vi "GUI_FilterWheels.vi"() -> ()   [LabVIEW 2020]
uses:
  Device Drivers/FilterWheels/posTypDef.ctl
  Device Drivers/FilterWheels/ModeTypDEf.ctl
panel:
  out "reference out":refnum<vi>
  out "#ofChannels":i32
  out "indecator ref array":refnum<vi>[](array[refnum])
  in  "time to wait (TCP) 2":i32=10
  in  "plot":bool=TRUE
  out "ratio(h)":bool
  out "fixsize":bool
  in  "shotnumber":i32
  out "error (h)":bool
  out "Device Name (h)":string="StagingDG645 1"
  in  "Main Tap":T1(tab)
  out "Description":string[](array[string])
  in  "ModeAll":T2
  in  "modeArray":T2[](array[typedef])
  out "Status 2":u32[](array[colorbox])
  out "Name":string[](array[string])
  in  "pos":T3[](array[typedef])
  out "device status":string
  out "local Port":u16=65427
  out "port or service name":u16=65426
  out "Remote Host":string="192.168.11.97"
  in  "timeout ms (slow resp)":i32=500
  in  "reset":bool
  out "All Devices (h)":string[](array[string])=["StagingDG645 1", "StagingDG645 2"]
  in  "time to wait (TCP)":i32=10
  out "error out":errorcluster
  out "connections (hidden)":variant[](array[variant])=[variant(refnum<k16> refnum), variant(refnum<k16> refnum)]
  in  "time to wait (main loop)":i32=10
  out "Data String":string="Amplitude.Ch AB,3.000000000000\r\nAmplitude.Ch CD,4.000000000000\r\nAmplitude.Ch EF,4.000000000000\r\nAmplitude.Ch GH,4.000000000000\r\nAmplitude.Ch T0,4.000000000000\r\nDelay.Ch A,0.000000000000\r\nDelay.Ch B,0.030000000000\r\nDelay.Ch C,0.000000000000\r\nDelay.Ch D,0.030000000000\r\nDelay.Ch E,0.000000000000\r\nDelay.Ch F,0.030000000000\r\nDelay.Ch G,0.000000000000\r\nDelay.Ch H,0.030000000000\r\nDelay.Ch T0,0.000000000000\r\nDelay.Ch T1,0.030000\r\nInhibit,Triggers\r\nLinked.Ch A,T0\r\nLinked.Ch B,A\r\nLinked.Ch C,T0\r\nLinked.Ch D,C\r\nLinked.Ch E,T0\r\nLinked.Ch F,E\r\nLinked.Ch G,T0\r\nLinked.Ch H,G\r\nLocalSavingPath,c:\\temp\r\nSave,off\r\nTrigger.ExecuteSingleShot,\r\nTrigger.Level,1.000000\r\nTrigger.Rate,10.000000\r\nTrigger.Source,External rising edges\r\ntimeout,0.000000\r\nPolarity.Ch AB,Positive\r\nPolarity.Ch CD,Positive\r\nPolarity.Ch EF,Positive\r\nPolarity.Ch GH,Positive\r\nPolarity.Ch T0,Positive\r\n"
  in  "Local Saving Path":path
  out "concatenated string":string
  out "subscriberString":string
  out "error message":string
  out "new data":bool
  out "Data Connection out":bool=TRUE
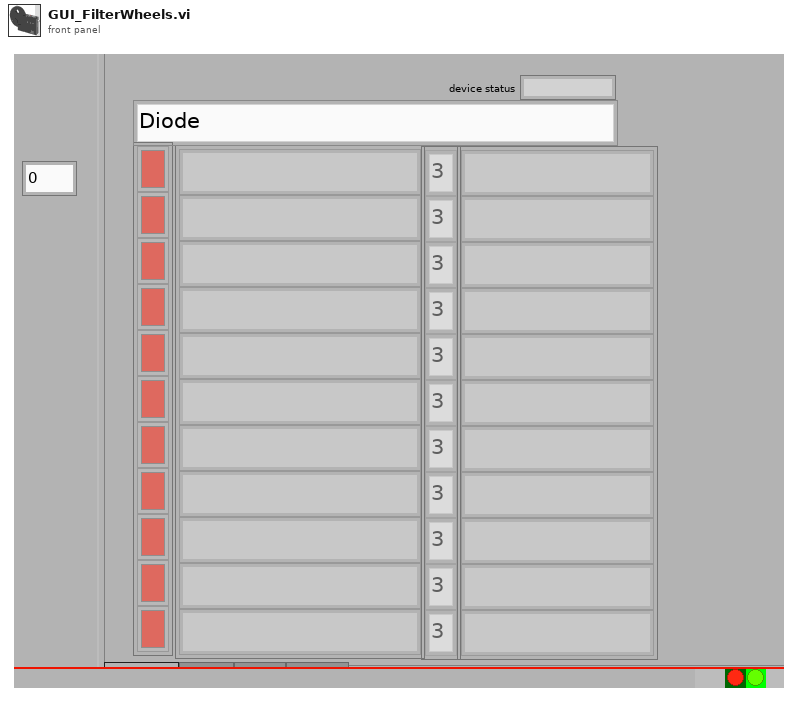
[diagram p1: front panel]
types:
  T1 = enum32{"All Channels", "Network", "Internal", "Advanced"}
  T2 = typedef "ModeTypDEf.ctl" = enum16{"Diode", "Low Power", "High Power", "undefined"}
  T3 = typedef "posTypDef.ctl" = enum16{"1", "2", "3", "4", "5", "6"}
  T4 = typedef "EventTypDef.ctl" = refnum<user-event>
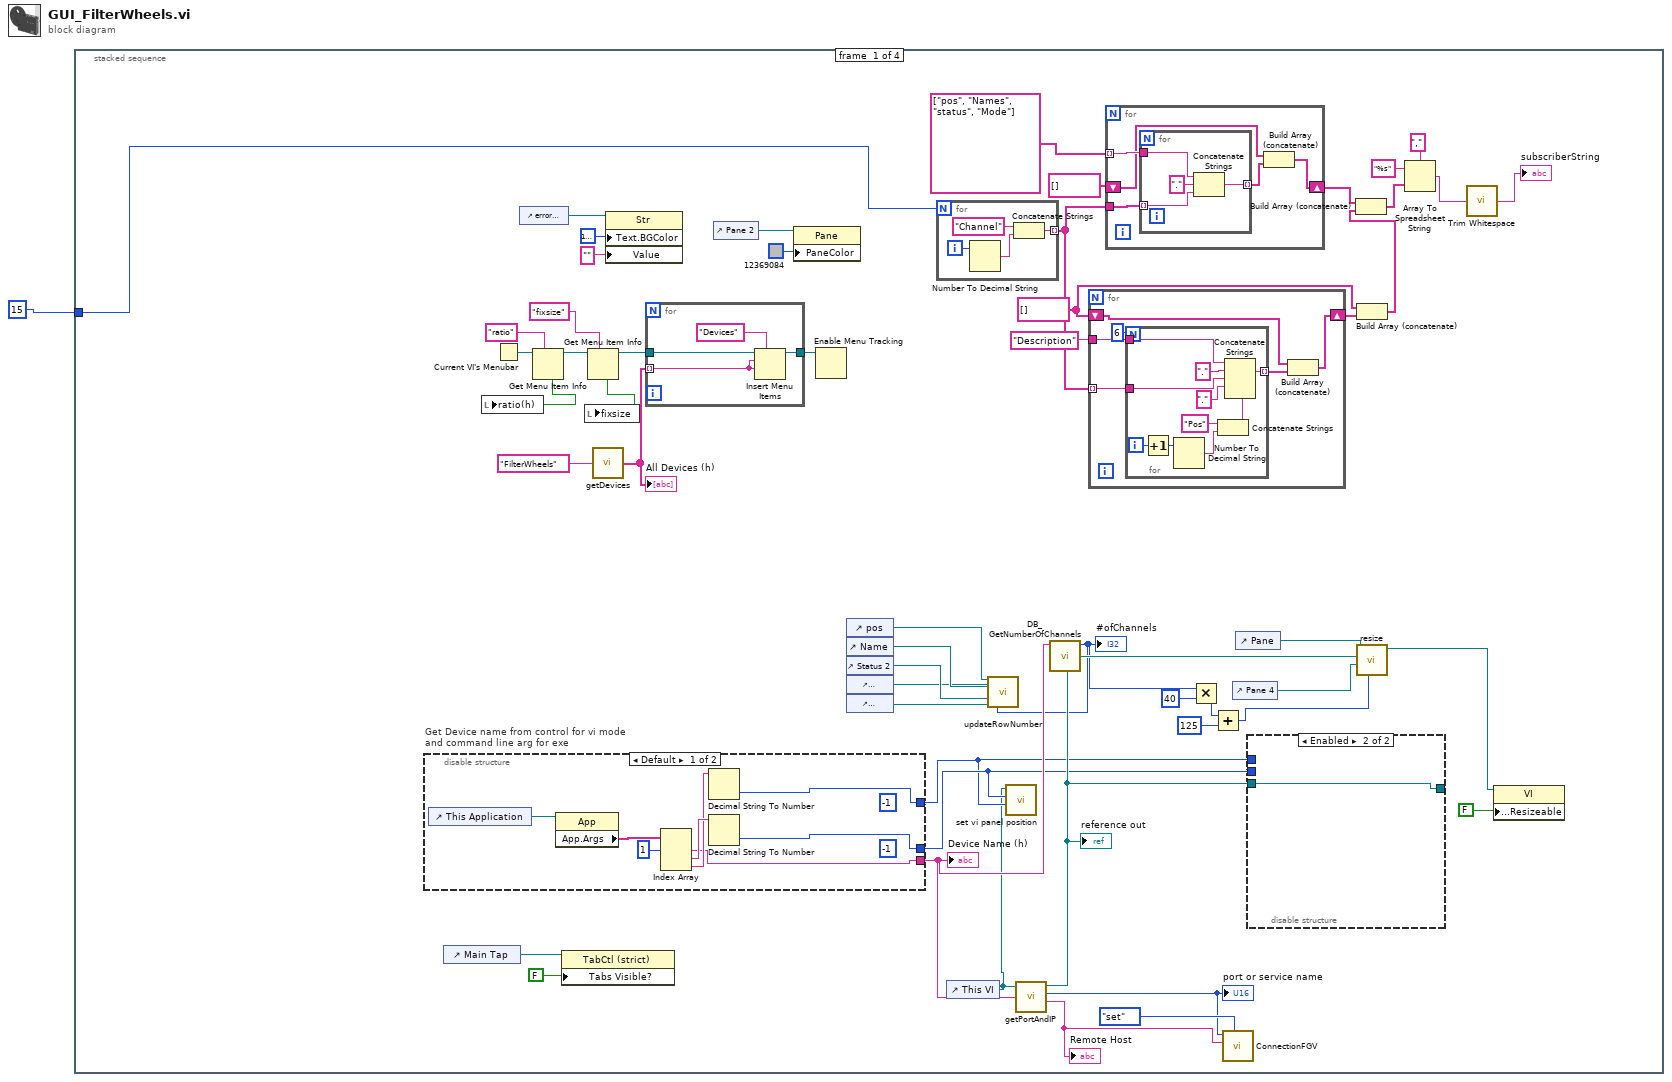
[diagram p0: block diagram]
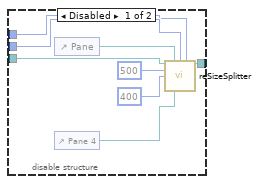
[diagram p2: hidden frame]
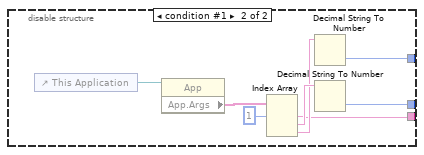
[diagram p3: hidden frame]
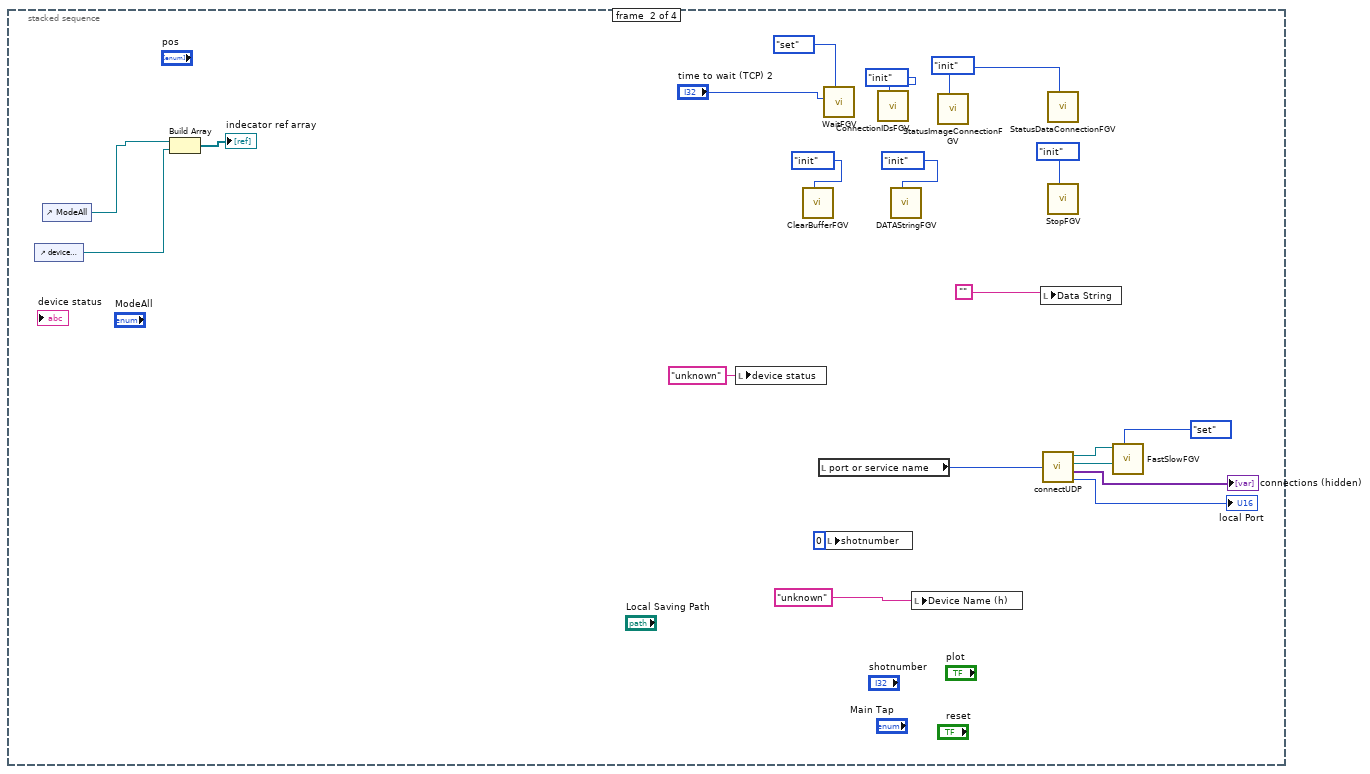
[diagram p4: hidden frame]
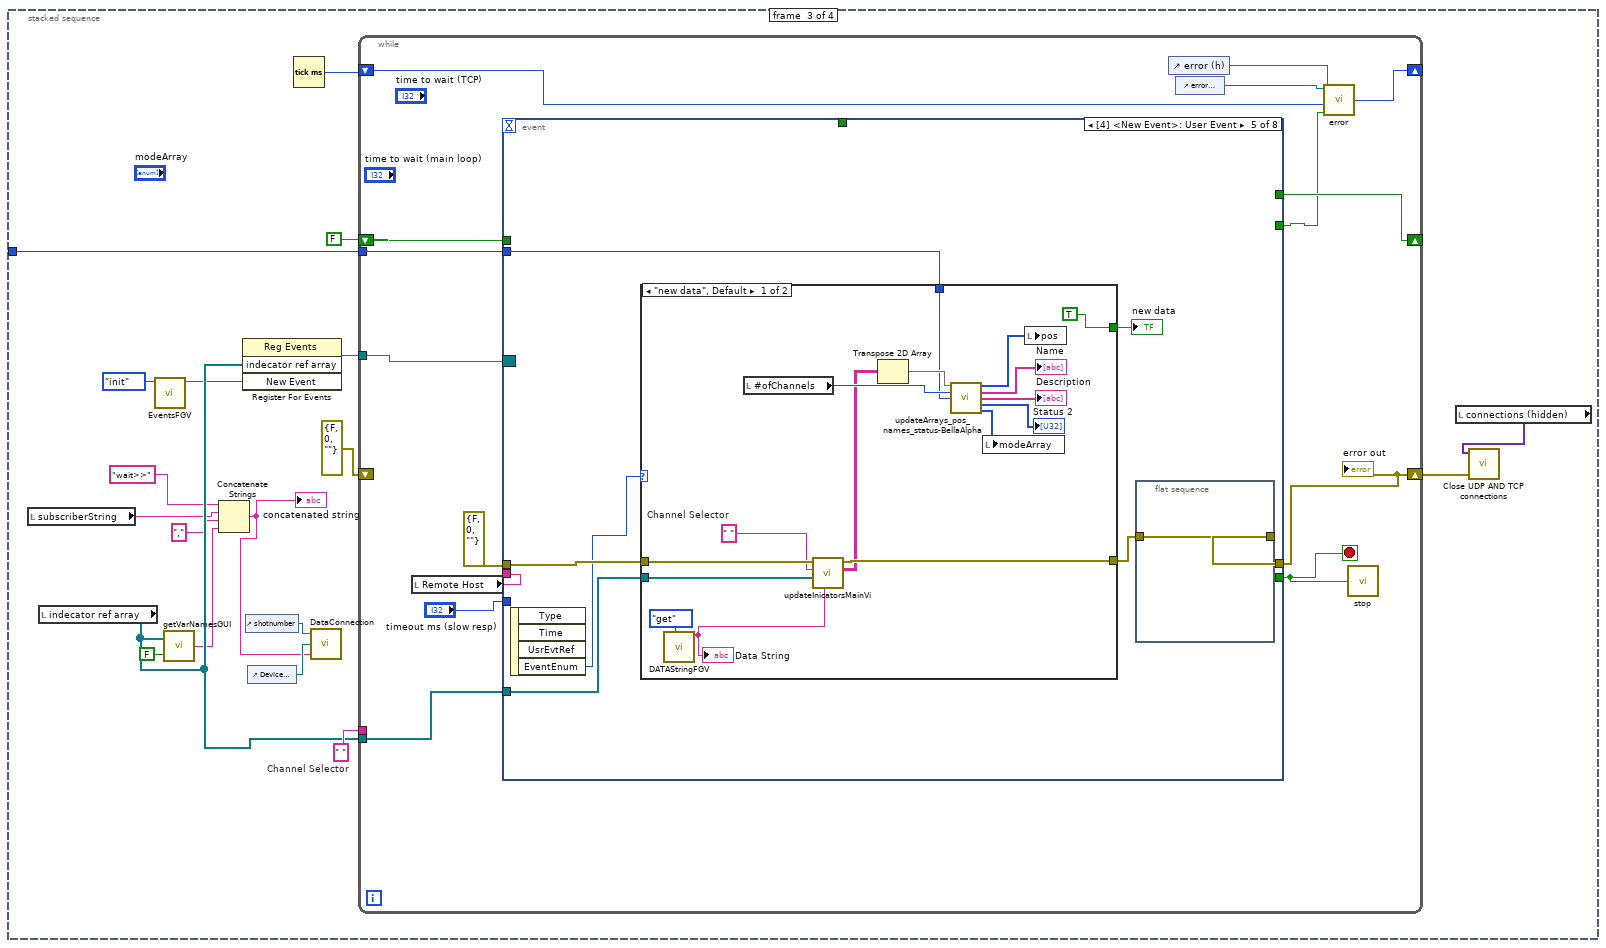
[diagram p5: hidden frame]
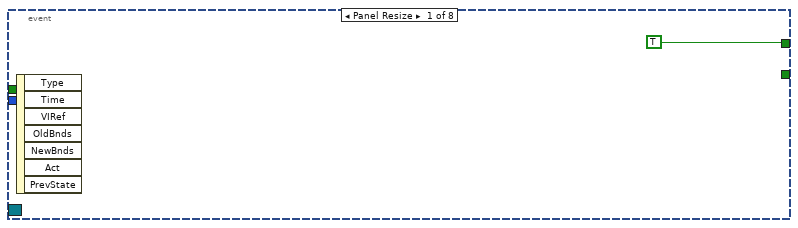
[diagram p6: hidden frame]
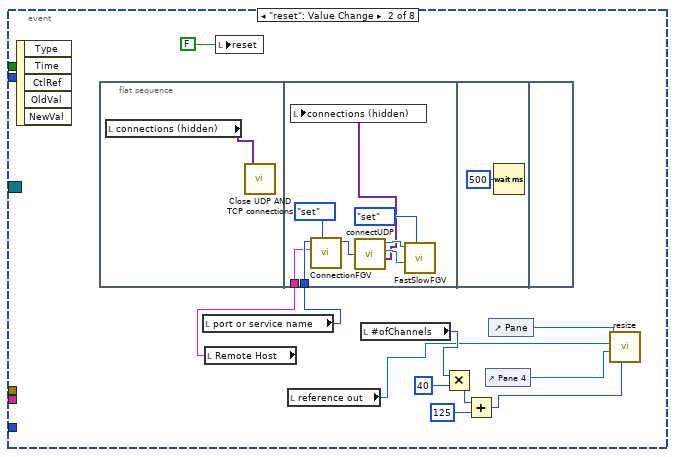
[diagram p7: hidden frame]
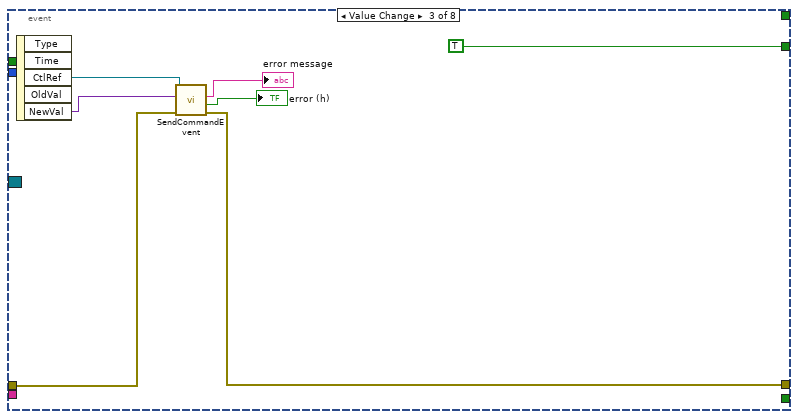
[diagram p8: hidden frame]
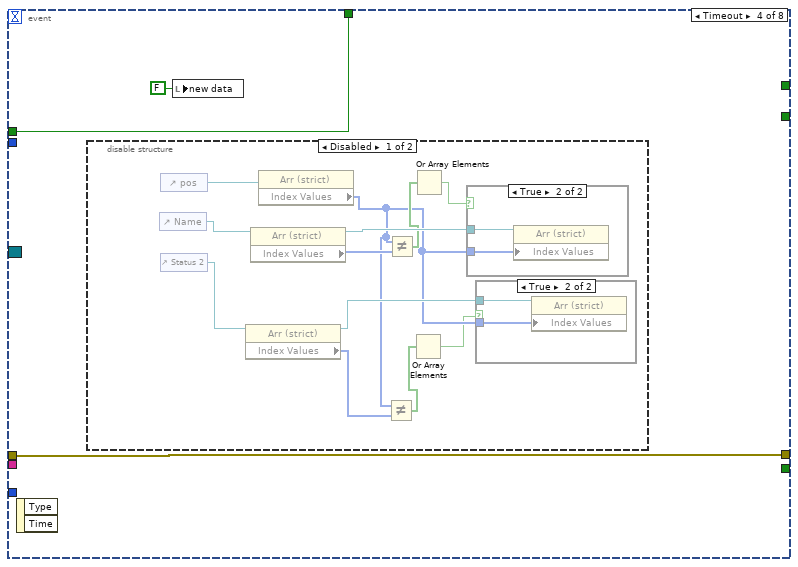
[diagram p9: hidden frame]
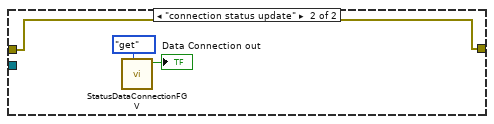
[diagram p13: hidden frame]
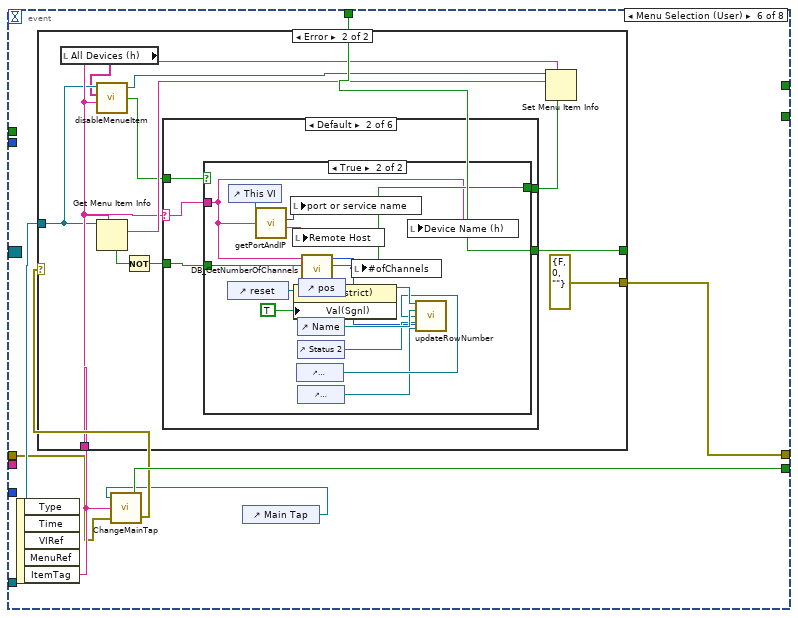
[diagram p14: hidden frame]
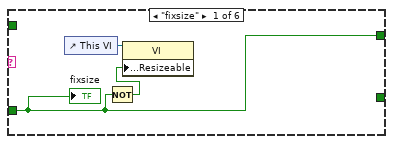
[diagram p16: hidden frame]
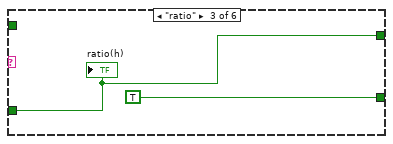
[diagram p18: hidden frame]
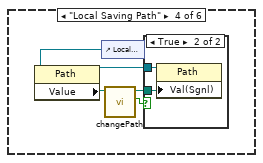
[diagram p19: hidden frame]
diagram:
  n1 = stacked-sequence {
    tunnel: 15 ("max channels") -> [w2 _ w133 _]
    frame #0 {
      w9 = string[] []
      n2 = disable-structure "Get Device name from control for vi mode\nand command line arg for exe" shown="Default" {
        disable-tunnel: [w97 w105] -> w33
        disable-tunnel: [w99 w108] -> w19
        disable-tunnel: [w100 w107] -> w18
        frame condition #0 (active) {
          (unwired) i16 -1 ("left")
          (unwired) i16 -1 ("left")
          n3 = control-ref of="This Application"() -> (w104:refnum<vi>)
          n4 = property class="App"(reference=w104) -> ("App.Args"=w98:string[])  [unwired: 1 in, 2 out]
          n5 = Index Array(array=w98, index #1=1 ("index")) -> (element #1=w97:string, element #2=w102:string, element #3=w101:string)  [unwired: 2 in]
          n6 = Decimal String To Number(string=w101) -> (number=w100:i32)  [unwired: 2 in, 1 out]
          n7 = Decimal String To Number(string=w102) -> (number=w99:i32)  [unwired: 2 in, 1 out]
        }
        frame condition #1 {
          n8 = control-ref of="This Application"() -> (w112:refnum<vi>)
          n9 = property class="App"(reference=w112) -> ("App.Args"=w106:string[])  [unwired: 1 in, 2 out]
          n10 = Index Array(array=w106, index #1=1 ("index")) -> (element #1=w105:string, element #2=w110:string, element #3=w109:string)  [unwired: 2 in]
          n11 = Decimal String To Number(string=w109) -> (number=w107:i32)  [unwired: 2 in, 1 out]
          n12 = Decimal String To Number(string=w110) -> (number=w108:i32)  [unwired: 2 in, 1 out]
        }
      }
      "Device Name (h)" <- w33
      n13 = control-ref of="Main Tap"() -> (w54:refnum<vi>)
      n14 = Current VI's Menubar() -> (w47:refnum<k9>)
      n15 = control-ref of="error message"() -> (w41:refnum<vi>)
      n16 = Get Menu Item Info(7:"ratio" ("item tag"), 11:w47) -> (3:w45:refnum<k9>, 4:w46:bool)  [unwired: 1 in, 5 out]
      n17 = local write "ratio(h)"(w46) -> ()
      n18 = property class="TabCtl (strict)"(reference=w54, "Tabs Visible?"=FALSE) -> ()  [unwired: 1 in, 2 out]
      n19 = Get Menu Item Info(7:"fixsize" ("item tag"), 11:w45) -> (3:w37:refnum<k9>, 4:w43:bool)  [unwired: 1 in, 5 out]
      n20 = local write "fixsize"(w43) -> ()
      n21 = call "getDevices.vi"("Device Class"="FilterWheels") -> ("All Devices"=w35:string[])
      "All Devices (h)" <- w35
      n22 = property class="Str"(reference=w41, "Text.BGColor"=u32 16777238, "Value"="") -> ()  [unwired: 1 in, 2 out]
      n23 = for {
        tunnel: w37 -> [w87]
        tunnel: [w86] -> w36
        tunnel: w35 -> [w84] mode=indexing
        n24 = Insert Menu Items(5:"Devices" ("menu tag"), 7:w84, 8:w84, 9:w87) -> (3:w86:refnum<k9>)  [unwired: 2 in, 2 out]
      }
      n25 = control-ref of="Pane 2"() -> (w39:refnum<vi>)
      n26 = property class="Pane"(reference=w39, "PaneColor"=u32 12369084) -> ()  [unwired: 1 in, 2 out]
      n27 = Enable Menu Tracking(4:w36) -> ()  [unwired: 2 in, 2 out]
      n28 = control-ref of="pos"() -> (w28:refnum<vi>)
      n29 = control-ref of="Name"() -> (w27:refnum<vi>)
      n30 = control-ref of="Status 2"() -> (w26:refnum<vi>)
      n31 = control-ref of="modeArray"() -> (w23:refnum<vi>)
      n32 = control-ref of="Description"() -> (w10:refnum<vi>)
      n33 = for {
        N: w2 -> [_]
        tunnel: [w80] -> w6 mode=indexing
        i -> [w83]
        n34 = Number To Decimal String(number=w83) -> (decimal integer string=w81:string)  [unwired: 1 in]
        n35 = Concatenate Strings("Channel" ("string"), w81) -> (w80:string)
      }
      n36 = control-ref of="This VI"() -> (w17:refnum<vi>)
      n37 = call "set vi panel position.vi"("top"=w18, "left"=w19, "This VI"=w17) -> ()  [unwired: 7 in, 2 out]
      n38 = call "getPortAndIP.vi"("Device Name"=w33, "This Vi"=w17) -> ("Remote Host"=w50:string, "port or service name"=w49:u16, "reference out"=w22:refnum<vi>)  [unwired: 2 in, 2 out]
      "port or service name" <- w49
      "Remote Host" <- w50
      "reference out" <- w22
      n39 = call "DB_GetNumberOfChannels.vi"("DeviceName"=w33) -> ("Numeric"=w20:i32)  [unwired: 9 in, 1 out]
      "#ofChannels" <- w20
      n40 = call "updateRowNumber.vi"("Array in"=w28, "Name"=w27, "modeArray 2"=w23, "Status 3"=w26, "Description"=w10, "No of channels"=w20) -> ()  [unwired: 10 in]
      n41 = for {
        tunnel: w6 -> [w59] mode=indexing
        tunnel: "Description" ("string") -> [w60]
        shift-right: [w55] -> w7
        shift-left: w9 -> [w57]
        n42 = for {
          N: 6 -> [_]
          tunnel: w60 -> [w70]
          tunnel: w59 -> [w69]
          tunnel: [w68] -> w56 mode=indexing
          i -> [w62]
          n43 = Increment(x=w62) -> (x+1=w61:i32)
          n44 = Number To Decimal String(number=w61) -> (decimal integer string=w65:string)  [unwired: 1 in]
          n45 = Concatenate Strings("Pos" ("string"), w65) -> (w63:string)
          n46 = Concatenate Strings(w70, "." ("string"), w69, "." ("string"), w63) -> (w68:string)
        }
        n47 = Build Array (concatenate)(w57, w56) -> (w55:string[])
      }
      n48 = for {
        tunnel: string[] ["pos", "Names", "status", "Mode"] -> [w74] mode=indexing
        tunnel: w6 -> [w75]
        shift-right: [w72] -> w4
        shift-left: string[] [] -> [w71]
        n49 = for {
          tunnel: w75 -> [w77] mode=indexing
          tunnel: w74 -> [w79]
          tunnel: [w76] -> w73 mode=indexing
          n50 = Concatenate Strings(w79, "." ("string"), w77) -> (w76:string)
        }
        n51 = Build Array (concatenate)(w71, w73) -> (w72:string[])
      }
      n52 = Multiply(x=w20, y=40) -> (x*y=w11:i32)
      n53 = Add(x=w11, y=125) -> (x+y=w12:i32)
      n54 = call "ConnectionFGV.vi"("command"=enum16{"get", "set", "init"}."set", "Remote Host in"=w50, "port or service name in"=w49) -> ()  [unwired: 7 in, 2 out]
      n55 = control-ref of="Pane 4"() -> (w15:refnum<vi>)
      n56 = control-ref of="Pane"() -> (w16:refnum<vi>)
      n57 = disable-structure shown="Enabled" {
        disable-tunnel: w19 -> [w94 _]
        disable-tunnel: w18 -> [w93 _]
        disable-tunnel: w22 -> [w91 w96]
        disable-tunnel: [w88 w96] -> _
        frame Disabled {
          n58 = control-ref of="Pane"() -> (w95:refnum<vi>)
          n59 = control-ref of="Pane 4"() -> (w92:refnum<vi>)
          n60 = call "reSizeSplitter.vi"("this vi"=w91, "pane"=w95, "left"=w94, "top"=w93, "Width"=u32 500, "Height"=u32 400, "pane2"=w92) -> ("reference out"=w88:refnum<vi>)  [unwired: 8 in]
        }
        frame Enabled {
        }
      }
      n61 = Build Array (concatenate)(w9, w7) -> (w5:string[])
      n62 = Build Array (concatenate)(w4, w5) -> (w3:string[])
      n63 = call "resize.vi"("Height"=w12, "Pane 4"=w15, "reference out 2"=w22, "Pane in"=w16) -> ("reference out"=w21:refnum<vi>)  [unwired: 7 in]
      n64 = Array To Spreadsheet String(delimiter (Tab)=",", array=w3, 3:"%s" ("format string")) -> (spreadsheet string=w25:string)
      n65 = call <vilib>:"Trim Whitespace.vi"("string"=w25) -> ("trimmed string"=→"subscriberString":string)  [unwired: 1 in]
      n66 = property class="VI"(reference=w21, "Front Panel.Resizeable"=FALSE ("Front Panel Window:Resizable")) -> ()  [unwired: 1 in, 2 out]
    }
    frame #1 {
      w125 = enum16{"get", "set", "init"}."init" ("Command")
      n67 = control-ref of="device status"() -> (w114:refnum<vi>)
      n68 = control-ref of="ModeAll"() -> (w115:refnum<vi>)
      n69 = Build Array(w115, w114) -> (→"indecator ref array":refnum<vi>[])
      n70 = local write "device status"("unknown" ("device status")) -> ()
      n71 = call "ClearBufferFGV.vi"("Command"=enum16{"set", "get", "init"}."init") -> ()  [unwired: 10 in, 1 out]
      n72 = local read "port or service name"() -> (w121:u16)
      n73 = call "WaitFGV.vi"("Command"=enum16{"get", "set", "init"}."set", "milliseconds to wait"="time to wait (TCP) 2") -> ()  [unwired: 9 in, 1 out]
      n74 = local write "shotnumber"(0 ("shotnumber")) -> ()
      n75 = call "ConnectionIDsFGV.vi"("Command"=enum16{"add", "get", "init"}."init") -> ()  [unwired: 10 in, 1 out]
      n76 = call "DATAStringFGV.vi"("Command"=enum16{"get", "set", "init"}."init") -> ()  [unwired: 9 in, 2 out]
      n77 = local write "Device Name (h)"("unknown" ("Device Name")) -> ()
      n78 = call "StatusImageConnectionFGV.vi"("Command"=w125) -> ()  [unwired: 10 in, 1 out]
      n79 = local write "Data String"("") -> ()
      n80 = call "connectUDP.vi"("port or service name NOT USED"=w121) -> ("fast ID (h)"=w120:refnum<k16>, "slow ID (h)"=w119:refnum<k16>, "connections (hidden)"=→"connections (hidden)":variant[], "local Port"=→"local Port":u16)
      n81 = call "StatusDataConnectionFGV.vi"("Command"=w125) -> ()  [unwired: 10 in, 1 out]
      n82 = call "StopFGV.vi"("Command"=enum16{"set", "get", "init"}."init") -> ()  [unwired: 9 in, 2 out]
      n83 = call "FastSlowFGV.vi"("Command"=enum16{"get", "set", "init"}."set", "slow ID"=w119, "fast ID"=w120) -> ()  [unwired: 7 in, 2 out]
    }
    frame #2 {
      w143 = " "  # Channel Selector
      n84 = local read "subscriberString"() -> (w138:string)
      n85 = local read "indecator ref array"() -> (w142:refnum<vi>[])
      n86 = call "EventsFGV.vi"("Command"=enum16{"get", "init"}."init") -> ("New Event"=w135:T4)  [unwired: 9 in, 1 out]
      n87 = call "getVarNamesGUI.vi"("start"=FALSE, "Array"=w142) -> ("String"=w137:string)
      n88 = Concatenate Strings("wait>>" ("string"), w138, "," ("string"), w137) -> (w140:string)
      "concatenated string" <- w140
      n89 = register-events(w142, w135) -> (reference out=w144:refnum<event-registration>)  [unwired: 2 in, 1 out]
      n90 = control-ref of="shotnumber"() -> (w146:refnum<vi>)
      n91 = control-ref of="Device Name (h)"() -> (w145:refnum<vi>)
      n92 = Tick Count (ms)() -> (millisecond timer value=w147:u32)
      n93 = call "DataConnection.vi"("Subscriber list"=w140, "Device Name (h)"=w145, "shotnumber"=w146) -> ()
      n94 = while {
        shift-right: [w154] -> w150
        shift-left: errorcluster {"status"=FALSE, "code"=0, "source"=""} ("error out") -> [_]
        tunnel: w142 -> [w155]
        shift-right: [w163] -> _
        shift-left: FALSE -> [w164]
        shift-right: [w162] -> _
        shift-left: w147 -> [w161]
        tunnel: w144 -> [w159]
        tunnel: w143 -> [_]
        tunnel: w133 -> [w152]
        stop <- w160 stop-if-true
        n95 = local read "Remote Host"() -> (w165:string)
        n96 = event shown="[4] <New Event>: User Event" {
          selector: w159 -> [_ _ _ _ _ _ _ _]
          dyn-events: _ -> [_ _ _ _ _ _ _ _]
          timeout: _ -> [_ _ _ _ _ _ _ _]
          tunnel: [_ _ w193 w198 w218 w243 w298 w322] -> w154
          tunnel: w165 -> [_ _ _ _ _ _ _ _]
          tunnel: "timeout ms (slow resp)" -> [_ _ _ _ _ _ _ _]
          tunnel: errorcluster {"status"=FALSE, "code"=0, "source"=""} ("error out") -> [_ _ w190 w198 w221 w244 w298 w322]
          tunnel: [_ _ TRUE _ _ _ TRUE TRUE] -> w153
          tunnel: [_ _ _ _ _ w249 _ _] -> w160
          tunnel: [_ _ _ w197 _ w246 _ _] -> _
          tunnel: w164 -> [_ _ _ w197 _ _ _ _]
          tunnel: [TRUE _ _ _ _ _ _ _] -> w163
          tunnel: w155 -> [_ _ _ _ w220 _ _ _]
          tunnel: w152 -> [_ _ _ _ w215 _ _ _]
          event Panel Resize {
            n97 = event-data() -> ()  [unwired: 1 in, 7 out]
          }
          event "reset": Value Change {
            n98 = event-data() -> ()  [unwired: 1 in, 5 out]
            n99 = flat-sequence {
              tunnel: w177 -> [w182]
              tunnel: w176 -> [w181]
              frame #0 {
                n100 = local read "connections (hidden)"() -> (w179:variant[])
                n101 = call "Close UDP AND TCP connections.vi"("appended array"=w179) -> ()  [unwired: 7 in]
              }
              frame #1 {
                n102 = call "ConnectionFGV.vi"("command"=enum16{"get", "set", "init"}."set", "Remote Host in"=w181, "port or service name in"=w182) -> ("port or service name out"=w186:u16)  [unwired: 7 in, 1 out]
                n103 = call "connectUDP.vi"("port or service name NOT USED"=w186) -> ("fast ID (h)"=w185:refnum<k16>, "slow ID (h)"=w184:refnum<k16>, "connections (hidden)"=w180:variant[])  [unwired: 1 out]
                n104 = local write "connections (hidden)"(w180) -> ()
                n105 = call "FastSlowFGV.vi"("Command"=enum16{"get", "set", "init"}."set", "slow ID"=w184, "fast ID"=w185) -> ()  [unwired: 7 in, 2 out]
              }
              frame #2 {
                n106 = Wait (ms)(milliseconds to wait=u32 500) -> ()  [unwired: 1 out]
              }
              frame #3 {
              }
            }
            n107 = local read "port or service name"() -> (w177:u16)
            n108 = local read "Remote Host"() -> (w176:string)
            n109 = local write "reset"(FALSE ("reset")) -> ()
            n110 = local read "reference out"() -> (w168:refnum<vi>)
            n111 = local read "#ofChannels"() -> (w169:i32)
            n112 = Multiply(x=w169, y=40) -> (x*y=w175:i32)
            n113 = Add(x=w175, y=125) -> (x+y=w174:i32)
            n114 = control-ref of="Pane 4"() -> (w171:refnum<vi>)
            n115 = control-ref of="Pane"() -> (w170:refnum<vi>)
            n116 = call "resize.vi"("Height"=w174, "Pane 4"=w171, "reference out 2"=w168, "Pane in"=w170) -> ()  [unwired: 7 in, 1 out]
          }
          event Value Change {
            n117 = event-data() -> ("CtlRef"=w195:refnum<vi>, "NewVal"=w194:variant)  [unwired: 1 in, 3 out]
            n118 = call "SendCommandEvent.vi"("error out 2"=w190, "NewVal"=w194, "CtlRef"=w195) -> ("error out"=w193:errorcluster, "error (h)"=→"error (h)":bool, "error message"=→"error message":string)  [unwired: 5 in, 1 out]
          }
          event Timeout {
            n119 = event-data() -> ()  [unwired: 1 in, 2 out]
            n120 = disable-structure shown="Disabled" {
              frame Disabled {
                n121 = control-ref of="Name"() -> (w207:refnum<vi>)
                n122 = control-ref of="pos"() -> (w210:refnum<vi>)
                n123 = control-ref of="Status 2"() -> (w209:refnum<vi>)
                n124 = property class="Arr (strict)"(reference=w209) -> (reference out=w208:refnum<vi>, "Index Values"=w201:u32[])  [unwired: 1 in, 1 out]
                n125 = property class="Arr (strict)"(reference=w207) -> (reference out=w206:refnum<vi>, "Index Values"=w205:u32[])  [unwired: 1 in, 1 out]
                n126 = property class="Arr (strict)"(reference=w210) -> ("Index Values"=w200:u32[])  [unwired: 1 in, 2 out]
                n127 = Not Equal?(x=w200, y=w201) -> (x != y?=w202:bool[])
                n128 = Not Equal?(x=w200, y=w205) -> (x != y?=w204:bool[])
                n129 = Or Array Elements(Boolean array=w202) -> (logical OR=w199:bool)
                n130 = Or Array Elements(Boolean array=w204) -> (logical OR=w203:bool)
                n131 = case shown="True" w203 {
                  tunnel: w206 -> [_ w214]
                  tunnel: w200 -> [_ w213]
                  frame False {
                  }
                  frame True {
                    n132 = property class="Arr (strict)"(reference=w214, "Index Values"=w213) -> ()  [unwired: 1 in, 2 out]
                  }
                }
                n133 = case shown="True" w199 {
                  tunnel: w208 -> [_ w212]
                  tunnel: w200 -> [_ w211]
                  frame False {
                  }
                  frame True {
                    n134 = property class="Arr (strict)"(reference=w212, "Index Values"=w211) -> ()  [unwired: 1 in, 2 out]
                  }
                }
              }
              frame Enabled {
              }
            }
            n135 = local write "new data"(FALSE ("new data")) -> ()
          }
          event User Event {
            n136 = event-data() -> ("EventEnum"=w217:enum16{"new data", "connection status update"})  [unwired: 1 in, 3 out]
            n137 = case shown="\"new data\", Default" w217 {
              tunnel: w221 -> [w238 w239]
              tunnel: [w237 w239] -> w219
              tunnel: w220 -> [w235 _]
              tunnel: [TRUE ("new data") _] -> w216
              tunnel: w215 -> [w223 _]
              frame "new data", Default {
                w236 = " "  # Channel Selector
                n138 = call "DATAStringFGV.vi"("Command"=enum16{"get", "set", "init"}."get") -> ("Data String out"=w233:string)  [unwired: 9 in, 1 out]
                "Data String" <- w233
                n139 = local read "#ofChannels"() -> (w231:i32)
                n140 = call "updateInicatorsMainVi.vi"("Data String out"=w233, "Array"=w235, "Channel Selector"=w236, "error in"=w238) -> ("name/data"=w227:string[][], "error out"=w237:errorcluster)  [unwired: 5 in, 1 out]
                n141 = Transpose 2D Array(2D array=w227) -> (transposed array=w226:string[][])
                n142 = call "updateArrays_pos_names_status-BellaAlpha.vi"("name/data 2"=w226, "#ofChannels"=w231, "max channels"=w223) -> ("pos"=w228:T3[], "Names"=→"Name":string[], "Description"=→"Description":string[], "Status"=→"Status 2":u32[], "Mode"=w232:T2[])  [unwired: 8 in]
                n143 = local write "modeArray"(w232) -> ()
                n144 = local write "pos"(w228) -> ()
              }
              frame "connection status update" {
                n145 = call "StatusDataConnectionFGV.vi"("Command"=enum16{"get", "set", "init"}."get") -> ("Data Connection out"=→"Data Connection out":bool)  [unwired: 10 in]
              }
            }
            "new data" <- w216
            n146 = flat-sequence {
              tunnel: w219 -> [w222]
              tunnel: [w222] -> w218
              frame #0 {
              }
            }
          }
          event Menu Selection (User) {
            n147 = event-data() -> ("MenuRef"=w245:refnum<k9>, "ItemTag"=w247:string)  [unwired: 1 in, 3 out]
            n148 = control-ref of="Main Tap"() -> (w242:refnum<vi>)
            n149 = call "ChangeMainTap.vi"("error in"=w244, "ItemTag"=w247, "reference"=w242) -> ("error out"=w248:errorcluster, "Boolean"=w249:bool)
            n150 = case shown="Error" w248 {
              selector: w248 -> [w250 _]
              tunnel: w245 -> [_ w256]
              tunnel: [_ w258] -> w246
              tunnel: w247 -> [_ w257]
              tunnel: [w250 errorcluster {"status"=FALSE, "code"=0, "source"=""} ("error IO")] -> w243
              frame No Error {
              }
              frame Error {
                n151 = local read "All Devices (h)"() -> (w251:string[])
                n152 = call "disableMenueItem.vi"("ItemTag"=w257, "All Devices (h)"=w251, "MenuRef"=w256) -> ("this is a Device(tag)"=w255:bool, "menu reference out"=w254:refnum<k9>)  [unwired: 1 in, 1 out]
                n153 = Get Menu Item Info(7:w257, 11:w256) -> (2:w260:string, 4:w261:bool)  [unwired: 1 in, 5 out]
                n154 = Not(x=w261) -> (.not. x?=w259:bool)
                n155 = case shown="Default" w257 {
                  selector: w257 -> [_ w267 _ _ _ _]
                  tunnel: w259 -> [w262 w265 w282 _ _ _]
                  tunnel: [_ _ TRUE _ _ _] -> w258
                  tunnel: w255 -> [_ w268 _ _ _ _]
                  tunnel: [w262 w266 w282 _ _ _] -> w253
                  frame "fixsize" {
                    n156 = control-ref of="This VI"() -> (w264:refnum<vi>)
                    n157 = Not(x=w262) -> (.not. x?=w263:bool)
                    n158 = property class="VI"(reference=w264, "Front Panel.Resizeable"=w263) -> ()  [unwired: 1 in, 2 out]
                    "fixsize" <- w262
                  }
                  frame Default {
                    n159 = case shown="True" w268 {
                      tunnel: w267 -> [_ w271]
                      tunnel: [_ w276] -> w266
                      tunnel: w265 -> [_ w276]
                      frame False {
                      }
                      frame True {
                        n160 = control-ref of="reset"() -> (w278:refnum<vi>)
                        n161 = control-ref of="This VI"() -> (w281:refnum<vi>)
                        n162 = call "getPortAndIP.vi"("Device Name"=w271, "This Vi"=w281) -> ("Remote Host"=w280:string, "port or service name"=w279:u16)  [unwired: 2 in, 3 out]
                        n163 = local write "port or service name"(w279) -> ()
                        n164 = local write "Remote Host"(w280) -> ()
                        n165 = property class="Bool (strict)"(reference=w278, "Val(Sgnl)"=TRUE ("Value (Signaling)")) -> ()  [unwired: 1 in, 2 out]
                        n166 = control-ref of="modeArray"() -> (w270:refnum<vi>)
                        n167 = control-ref of="Name"() -> (w274:refnum<vi>)
                        n168 = control-ref of="Status 2"() -> (w273:refnum<vi>)
                        n169 = control-ref of="Description"() -> (w269:refnum<vi>)
                        n170 = control-ref of="pos"() -> (w275:refnum<vi>)
                        n171 = call "DB_GetNumberOfChannels.vi"("DeviceName"=w271) -> ("Numeric"=w272:i32)  [unwired: 9 in, 1 out]
                        n172 = local write "#ofChannels"(w272) -> ()
                        n173 = local write "Device Name (h)"(w271) -> ()
                        n174 = call "updateRowNumber.vi"("Array in"=w275, "Name"=w274, "modeArray 2"=w270, "Status 3"=w273, "Description"=w269, "No of channels"=w272) -> ()  [unwired: 10 in]
                      }
                    }
                  }
                  frame "ratio" {
                    "ratio(h)" <- w282
                  }
                  frame "Local Saving Path" {
                    n175 = control-ref of="Local Saving Path"() -> (w284:refnum<vi>)
                    n176 = property class="Path"(reference=w284) -> (reference out=w287:refnum<vi>, "Value"=w288:path)  [unwired: 1 in, 1 out]
                    n177 = call "changePath.vi"("Local Saving in (h)"=w288) -> ("change (h)"=w286:bool, "Local Saving out (h)"=w285:path)  [unwired: 9 in]
                    n178 = case shown="True" w286 {
                      tunnel: w287 -> [_ w290]
                      tunnel: w285 -> [_ w289]
                      frame False {
                      }
                      frame True {
                        n179 = property class="Path"(reference=w290, "Val(Sgnl)"=w289) -> ()  [unwired: 1 in, 2 out]
                      }
                    }
                  }
                  frame "reset" {
                    n180 = control-ref of="reset"() -> (w292:refnum<vi>)
                    n181 = property class="Bool (strict)"(reference=w292, "Val(Sgnl)"=TRUE ("Value (Signaling)")) -> ()  [unwired: 1 in, 2 out]
                  }
                  frame "clear" {
                    n182 = control-ref of="reset"() -> (w294:refnum<vi>)
                    n183 = property class="Bool (strict)"(reference=w294, "Val(Sgnl)"=TRUE ("Value (Signaling)")) -> ()  [unwired: 1 in, 2 out]
                  }
                }
                n184 = Set Menu Item Info(6:w253, 7:w257, 10:w260, 11:w254) -> ()  [unwired: 3 in, 2 out]
              }
            }
          }
          event "pos": Value Change {
            n185 = event-data() -> ("OldVal"=w316:T3[], "NewVal"=w313:T3[])  [unwired: 1 in, 3 out]
            n186 = Not Equal?(x=w316, y=w313) -> (x != y?=w315:bool[])
            n187 = Search 1D Array(1D array=w315, element=TRUE) -> (index of element=w306:i32)  [unwired: 1 in]
            n188 = Number To Decimal String(number=w306) -> (decimal integer string=w305:string)  [unwired: 1 in]
            n189 = Index Array(array=w313, index=w306) -> (element=w296:T3)
            n190 = To Long Integer(number=w296) -> (32bit integer=w295:i32)
            n191 = call "ConnectionFGV.vi"("command"=enum16{"get", "set", "init"}."get") -> ("Remote Host out"=w311:string, "port or service name out"=w312:u16)  [unwired: 9 in]
            n192 = Increment(x=w295) -> (x+1=w299:i32)
            n193 = Number To Decimal String(number=w299) -> (decimal integer string=w303:string)  [unwired: 1 in]
            n194 = Concatenate Strings("set", "pos.Channel" ("string"), w305, ">>" ("string"), w303) -> (w309:string)
            n195 = call "sendCommandAndListen.vi"("command in"=w309, "error in"=w298, "Remote Host"=w311, "port or service name"=w312) -> ("error"=w301:bool, "error message"=w302:string, "error out"=w300:errorcluster)  [unwired: 8 in, 5 out]
            n196 = local write "error message"(w302) -> ()
            n197 = call <vilib>:"Clear Errors.vi"("error in (no error)"=w300) -> ()  [unwired: 5 in, 2 out]
            n198 = local write "error (h)"(w301) -> ()
          }
          event "modeArray": Value Change {
            n199 = event-data() -> ("OldVal"=w338:T2[], "NewVal"=w335:T2[])  [unwired: 1 in, 3 out]
            n200 = Not Equal?(x=w338, y=w335) -> (x != y?=w337:bool[])
            n201 = Search 1D Array(1D array=w337, element=TRUE) -> (index of element=w328:i32)  [unwired: 1 in]
            n202 = Number To Decimal String(number=w328) -> (decimal integer string=w327:string)  [unwired: 1 in]
            n203 = Index Array(array=w335, index=w328) -> (element=w319:T2)
            n204 = call "ConnectionFGV.vi"("command"=enum16{"get", "set", "init"}."get") -> ("Remote Host out"=w333:string, "port or service name out"=w334:u16)  [unwired: 9 in]
            n205 = call <userlib>:"Get Strings from Enum__ogtk.vi"("Enum"=ModeTypDEf."Low Power" ("Mode")) -> ("Enum Strings"=w320:string[])  [unwired: 7 in, 3 out]
            n206 = Index Array(array=w320, index=w319) -> (element=w318:string)
            n207 = Concatenate Strings("set", "Mode.Channel" ("string"), w327, ">>" ("string"), w318) -> (w331:string)
            n208 = call "sendCommandAndListen.vi"("command in"=w331, "error in"=w322, "Remote Host"=w333, "port or service name"=w334) -> ("error"=w324:bool, "error message"=w325:string, "error out"=w323:errorcluster)  [unwired: 8 in, 5 out]
            n209 = local write "error message"(w325) -> ()
            n210 = call <vilib>:"Clear Errors.vi"("error in (no error)"=w323) -> ()  [unwired: 5 in, 2 out]
            n211 = local write "error (h)"(w324) -> ()
          }
        }
        "error out" <- w154
        n212 = control-ref of="error (h)"() -> (w156:refnum<vi>)
        n213 = control-ref of="error message"() -> (w157:refnum<vi>)
        n214 = call "error.vi"("Boolean"=w153, "millisecond timer value"=w161, "reference"=w156, "error message"=w157) -> ("millisecond timer value 2"=w162:u32)
        n215 = call "stop.vi"("Boolean"=w160) -> ()
      }
      n216 = local read "connections (hidden)"() -> (w149:variant[])
      n217 = call "Close UDP AND TCP connections.vi"("error in"=w150, "appended array"=w149) -> ()  [unwired: 6 in]
    }
    frame #3 {
      n218 = control-ref of="Main  Control"() -> (w340:refnum<vi>)
      n219 = property class="TabCtl (strict)"(reference=w340, "Tabs Visible?"=TRUE) -> ()  [unwired: 1 in, 2 out]
      n220 = property class="TabCtl (strict)"(reference=w340, "Tab Location"=enum32{"Top", "Bottom", "Left", "Right"}."Bottom") -> ()  [unwired: 1 in, 2 out]
      n221 = flat-sequence {
        frame #0 {
          n222 = Wait (ms)(milliseconds to wait=u32 0) -> ()  [unwired: 1 out]
        }
        frame #1 {
        }
        frame #2 {
          n223 = control-ref of="This VI"() -> (w345:refnum<vi>)
          n224 = case shown="True" FALSE {
            tunnel: w345 -> [w346 w349]
            tunnel: [w346 w347] -> w344
            frame False {
            }
            frame True {
              n225 = property class="VI" props=["Front Panel.Open"](reference=w349) -> (reference out=w348:refnum<vi>)  [unwired: 1 in, 2 out]
              n226 = invoke class="VI" method="FP.Close"(reference=w348) -> (reference out=w347:refnum<vi>)  [unwired: 2 in, 2 out]
            }
          }
          n227 = Close Reference(reference=w344) -> ()  [unwired: 1 in, 1 out]
        }
      }
    }
  }
